vi "Is Point In Box.vi"(10 "AABB":T1, 11 "Point":refnum<class "Vector 2D.lvclass">) -> (3 "In Box?":bool)   [LabVIEW 2021, in "Collision.lvlib"]
uses:
  Collision.lvlib
  Vector 2D/Vector 2D.lvclass
  Vector 2D/Vector 2D.lvclass/Vector 2D.ctl
  Utility/Typedef/Axis Aligned Bounding Box.ctl
  Utility/Utility.lvlib
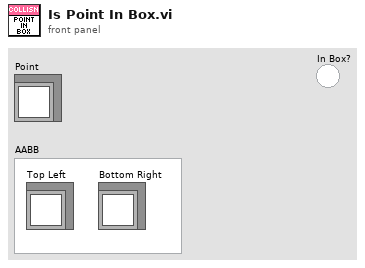
[diagram p1: front panel]
types:
  T1 = typedef "Utility.lvlib/Axis Aligned Bounding Box.ctl" = cluster{"Top Left":refnum<class "Vector 2D.lvclass">, "Bottom Right":refnum<class "Vector 2D.lvclass">}
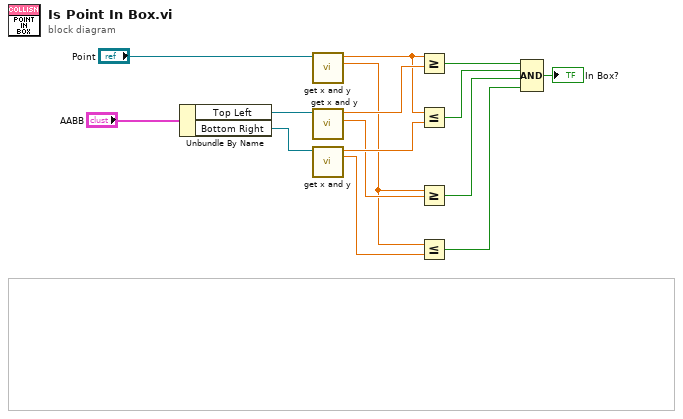
[diagram p0: block diagram]
diagram:
  n1 = Unbundle By Name("AABB") -> ("Top Left"=w14:refnum<class "Vector 2D.lvclass">, "Bottom Right"=w13:refnum<class "Vector 2D.lvclass">)
  n2 = call "get x and y.vi"("Vector 2D in"="Point") -> ("y"=w7:sgl, "x"=w10:sgl)  [unwired: 9 in]
  n3 = call "get x and y.vi"("Vector 2D in"=w14) -> ("y"=w8:sgl, "x"=w11:sgl)  [unwired: 9 in]
  n4 = call "get x and y.vi"("Vector 2D in"=w13) -> ("y"=w6:sgl, "x"=w9:sgl)  [unwired: 9 in]
  n5 = Greater Or Equal?(x=w10, y=w11) -> (x >= y?=w5:bool)
  n6 = Less Or Equal?(x=w10, y=w9) -> (x <= y?=w4:bool)
  n7 = Greater Or Equal?(x=w7, y=w8) -> (x >= y?=w3:bool)
  n8 = Less Or Equal?(x=w7, y=w6) -> (x <= y?=w2:bool)
  n9 = Compound Arithmetic op=AND(w5, w4, w3, w2) -> (→"In Box?":bool)
